vi "SRDG535.evt Call Get Output.vi"(0 "i ref in":refnum<vi>, 4 "output":u16(ring) items=["T0", "A", "B", "AB", "C", "D", "CD"], 5 "error IO":errorcluster, 6 "Generator Instance":string="N/A") -> (14 "i ref out":refnum<vi>, 19 "error out":errorcluster)   [LabVIEW 2014, in "SRDG535.lvlib"]
doc: "This VI sends a simple event call."
uses:
  SRDG535.lvlib
  CS_Core/CSSystem/CoreLib/CoreLib.short 2 byte array.vi
  CS_Core/CSSystem/CoreLib/CoreLib.lvlib
  CS_Core/BaseProcess/BaseProcess.lvlib
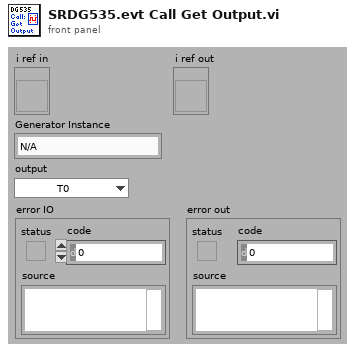
[diagram p1: front panel]
types:
  T1 = typedef "CoreDefs.rawDataType.ctl" = i8[]
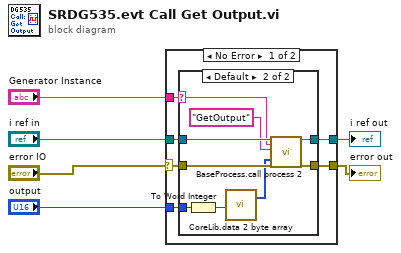
[diagram p0: block diagram]
diagram:
  n1 = case shown="No Error" "error IO" {
    selector: "error IO" -> [w12 w24]
    tunnel: "Generator Instance" -> [w7 _]
    tunnel: [w11 w24] -> w6
    tunnel: [w9 w25] -> w5
    tunnel: "output" -> [w8 _]
    tunnel: "i ref in" -> [w10 w25]
    frame No Error {
      n2 = case shown="Default" w7 {
        selector: w7 -> [_ w16]
        tunnel: w12 -> [w13 w23]
        tunnel: [w13 w22] -> w11
        tunnel: w10 -> [w14 w21]
        tunnel: [w14 w20] -> w9
        tunnel: w8 -> [_ w18]
        frame "", "N/A" {
        }
        frame Default {
          n3 = To Word Integer(number=w18) -> (16bit integer=w17:i16)
          n4 = call-poly "CoreLib.data 2 byte array.vi"("i16"=w17) -> ("byteArray out"=w15:T1)  [unwired: 18 in]
          n5 = call "BaseProcess.call process 2.vi"("i ref in"=w21, "Object"=w16, "Selector"="GetOutput", "Data"=w15, "error in (no error)"=w23) -> ("i ref out"=w20:refnum<vi>, "error out"=w22:errorcluster)  [unwired: 13 in]
        }
      }
    }
    frame Error {
    }
  }
  "error out" <- w6
  "i ref out" <- w5
